vi "num to string example.vi"() -> ()   [LabVIEW 2012]
panel:
  out "concatenated string":string
  out "string":string
  out "unsigned byte array":u8[](array[numeric]) format="%01x"
  in  "stop":bool
  in  "value (0)":i32=1234
  out "output string":string
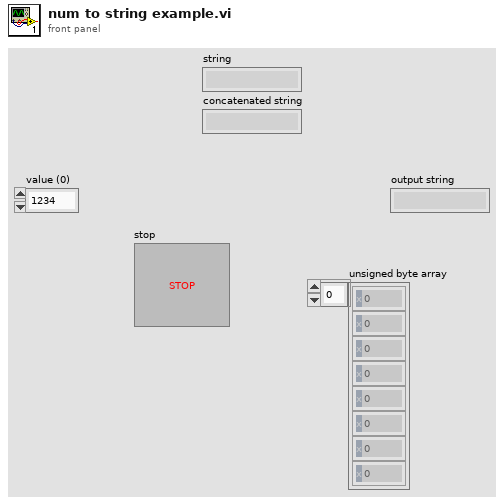
[diagram p1: front panel]
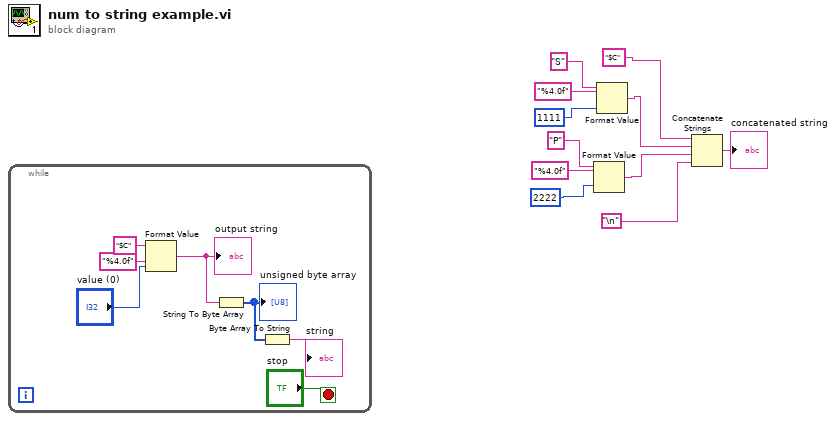
[diagram p0: block diagram]
diagram:
  n1 = while {
    stop <- "stop" stop-if-true
    n2 = Format Value(string ("")="$C", format string="%4.0f", value (0)="value (0)") -> (output string=w14:string)
    "output string" <- w14
    n3 = String To Byte Array(string=w14) -> (unsigned byte array=w13:u8[])
    "unsigned byte array" <- w13
    n4 = Byte Array To String(unsigned byte array=w13) -> (string=→"string":string)
  }
  n5 = Format Value(string ("")="P", format string="%4.0f", value (0)=2222) -> (output string=w3:string)
  n6 = Format Value(string ("")="S", format string="%4.0f", value (0)=1111) -> (output string=w4:string)
  n7 = Concatenate Strings("$C", w4, w3, "\n") -> (→"concatenated string":string)
